vi "LoadLearnFilter.vi"() -> ()   [LabVIEW 2016]
panel:
  out "den_Q3":dbl[](array[numeric])
  out "sum F":dbl[](array[numeric])
  out "num_G3":dbl[](array[numeric])
  out "num_G2":dbl[](array[numeric])
  out "num_G1":dbl[](array[numeric])
  out "Q2":cluster{i32, dbl[], dbl[]}
  out "den_Q2":dbl[](array[numeric])
  out "den_N1":dbl[](array[numeric])
  out "num_N1":dbl[](array[numeric])
  out "N3":cluster{i32, dbl[], dbl[]}
  out "den_N3":dbl[](array[numeric])
  out "num_N3":dbl[](array[numeric])
  out "N2":cluster{i32, dbl[], dbl[]}
  out "den_N2":dbl[](array[numeric])
  out "num_N2":dbl[](array[numeric])
  out "N1":cluster{i32, dbl[], dbl[]}
  out "num_Q3":dbl[](array[numeric])
  out "num_Q2":dbl[](array[numeric])
  out "num_F1":dbl[](array[numeric])
  out "num_F2":dbl[](array[numeric])
  out "num_Q1":dbl[](array[numeric])
  out "num_F3":dbl[](array[numeric])
  out "Joint 3 FIlter":dbl[][](graph)
  out "Joint 2 Filters":dbl[][](graph)
  out "Joint 1 Filters":dbl[][](graph)
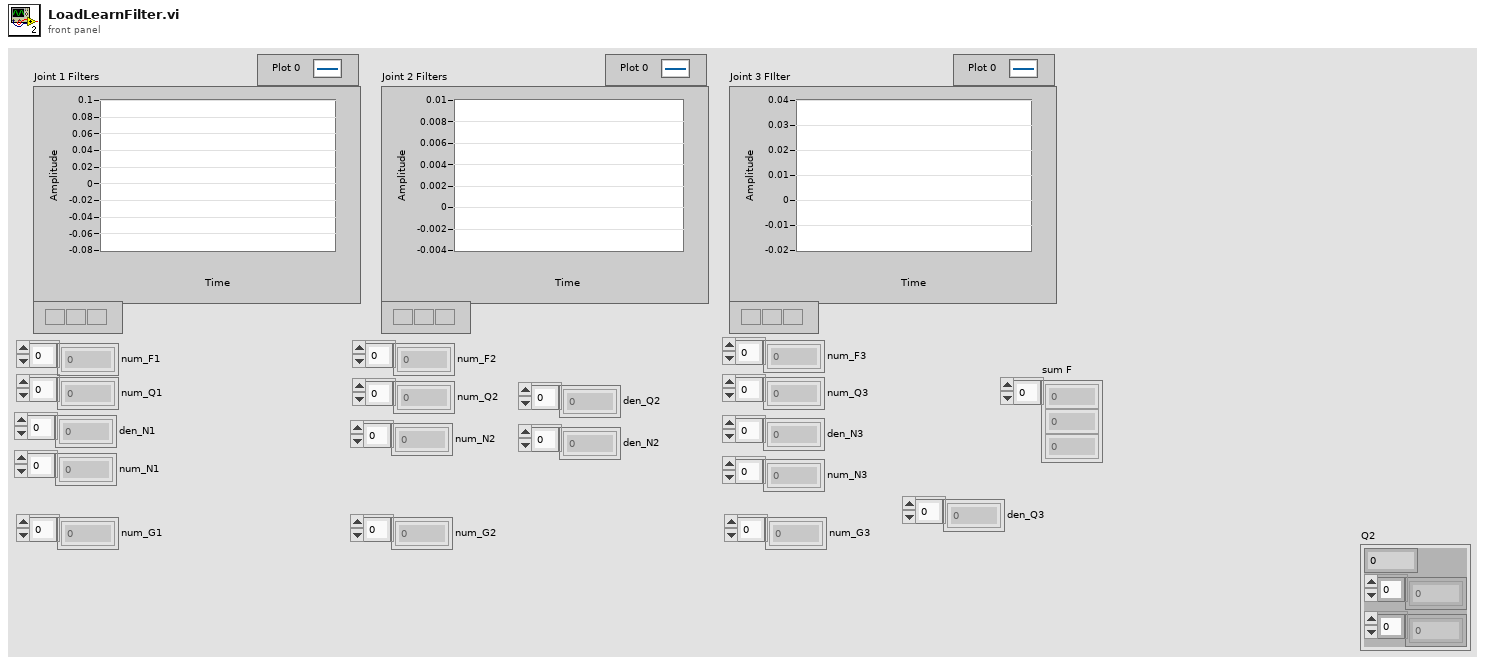
[diagram p1: front panel]
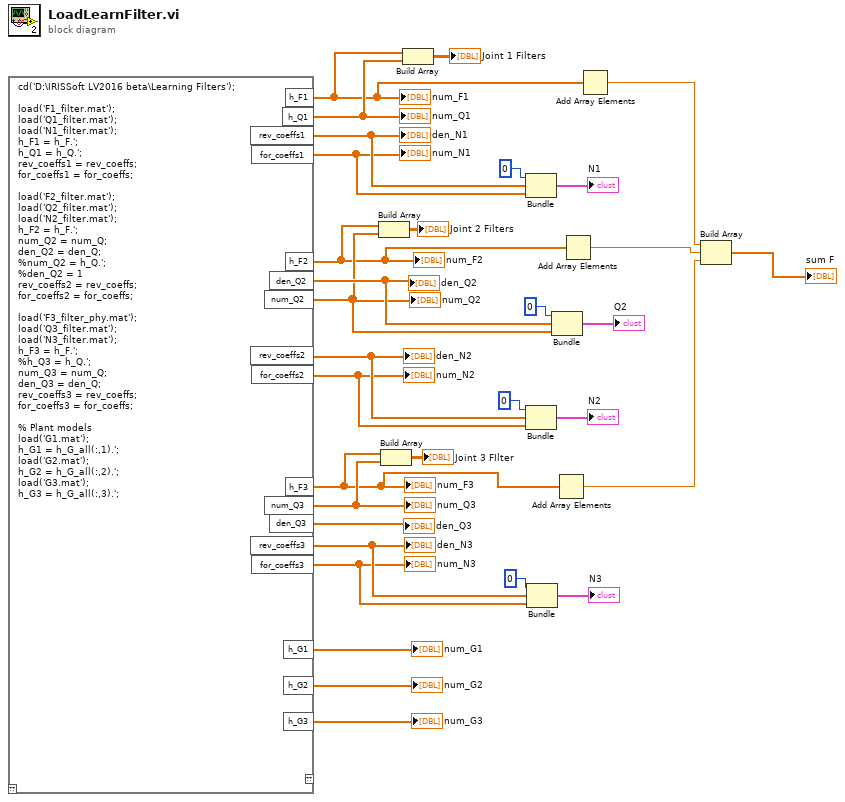
[diagram p0: block diagram]
diagram:
  n1 = script code="cd('D:\\IRISSoft LV2016 beta\\Learning Filters');\n\nload('F1_filter.mat'); \nload('Q1_filter.mat');\nload('N1_filter.mat');\nh_F1 = h_F.';\nh_Q1 = h_Q.';\nrev_coeffs1 = rev_coeffs;\nfor_coeffs1 = for_coeffs;\n\nload('F2_filter.mat'); \nload('Q2_filter.mat');\nload('N2_filter.mat');\nh_F2 = h_F.'; \nnum_Q2 = num_Q;\nden_Q2 = den_Q;\n%num_Q2 = h_Q.';\n%den_Q2 = 1\nrev_coeffs2 = rev_coeffs;\nfor_coeffs2 = for_coeffs;\n\nload('F3_filter_phy.mat');\nload('Q3_filter.mat');\nload('N3_filter.mat');\nh_F3 = h_F.'; \n%h_Q3 = h_Q.';\nnum_Q3 = num_Q;\nden_Q3 = den_Q;\nrev_coeffs3 = rev_coeffs;\nfor_coeffs3 = for_coeffs;\n\n% Plant models\nload('G1.mat');\nh_G1 = h_G_all(:,1).';\nload('G2.mat');\nh_G2 = h_G_all(:,2).';\nload('G3.mat');\nh_G3 = h_G_all(:,3).';"() -> ("h_F3"=w6:dbl[], "h_Q1"=w9:dbl[], "h_F2"=w7:dbl[], "h_F1"=w8:dbl[], "num_Q2"=w13:dbl[], "num_Q3"=w30:dbl[], "rev_coeffs1"=w18:dbl[], "for_coeffs1"=w17:dbl[], "rev_coeffs2"=w24:dbl[], "for_coeffs2"=w23:dbl[], "rev_coeffs3"=w20:dbl[], "for_coeffs3"=w19:dbl[], "den_Q2"=w14:dbl[], "h_G1"=→"num_G1":dbl[], "h_G2"=→"num_G2":dbl[], "h_G3"=→"num_G3":dbl[], "den_Q3"=→"den_Q3":dbl[])  [unwired: 1 in, 1 out]
  "num_F3" <- w6
  "num_Q1" <- w9
  "num_F2" <- w7
  "num_F1" <- w8
  "num_Q2" <- w13
  "num_Q3" <- w30
  "num_N2" <- w23
  "den_N2" <- w24
  "num_N3" <- w19
  "den_N3" <- w20
  "num_N1" <- w17
  "den_N1" <- w18
  "den_Q2" <- w14
  n2 = Build Array(w7, w13) -> (→"Joint 2 Filters":dbl[][])
  n3 = Build Array(w6, w30) -> (→"Joint 3 FIlter":dbl[][])
  n4 = Build Array(w8, w9) -> (→"Joint 1 Filters":dbl[][])
  n5 = Bundle(0, w18, w17) -> (→"N1":cluster{i32, dbl[], dbl[]})  [unwired: 1 in]
  n6 = Bundle(0, w24, w23) -> (→"N2":cluster{i32, dbl[], dbl[]})  [unwired: 1 in]
  n7 = Bundle(0, w20, w19) -> (→"N3":cluster{i32, dbl[], dbl[]})  [unwired: 1 in]
  n8 = Bundle(0, w14, w13) -> (→"Q2":cluster{i32, dbl[], dbl[]})  [unwired: 1 in]
  n9 = Add Array Elements(numeric array=w6) -> (sum=w2:dbl)
  n10 = Add Array Elements(numeric array=w7) -> (sum=w3:dbl)
  n11 = Add Array Elements(numeric array=w8) -> (sum=w4:dbl)
  n12 = Build Array(w4, w3, w2) -> (→"sum F":dbl[])
